vi "GetBeamPrams.vi"(4 "data":dbl[][](array[numeric]) format="%.2f", 7 "ycoords":dbl[](array[numeric]) format="%.2f", 8 "x coords":dbl[](array[numeric]) format="%.2f") -> (0 "3 dB beamwidth (cm)":dbl format="%.4f", 1 "lateral pressure (y)":cluster{"output":dbl[], "output":dbl[]}(graph), 2 "axial peak (cm)":dbl format="%.2f", 3 "axial pressure (z)":cluster{dbl[], "output":dbl[]}(graph))   [LabVIEW 2022 SP3]
uses:
  <vilib>/Utility/file.llb/Read From Spreadsheet File (DBL).vi
  <vilib>/Utility/file.llb/Write To Spreadsheet File (DBL).vi
  <vilib>/Analysis/NI_AALBase.lvlib
panel:
  in  "Case Constant\n(See Context Help)":bool=TRUE
  in  "save main axis":bool
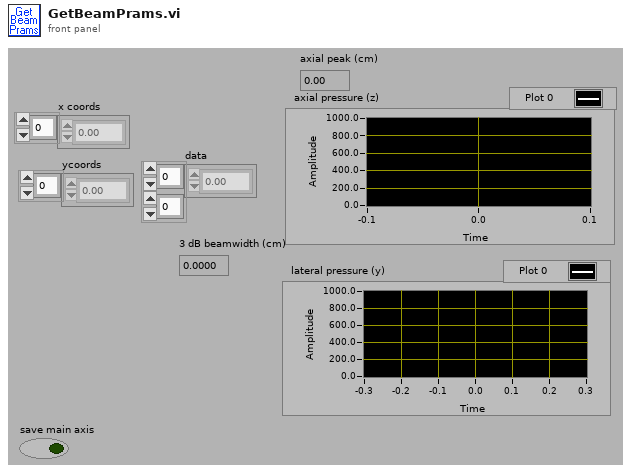
[diagram p1: front panel]
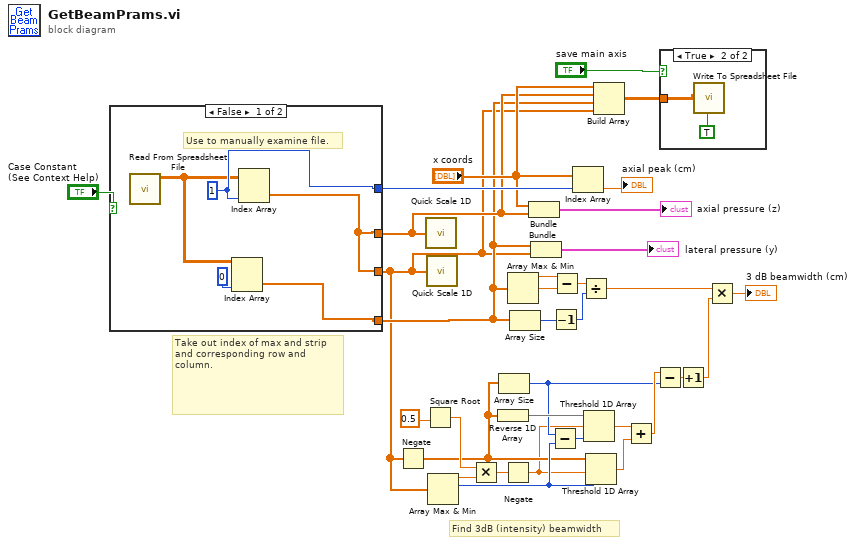
[diagram p0: block diagram]
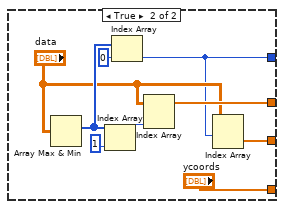
[diagram p3: hidden frame]
diagram:
  # "Take out index of max and strip and corresponding row and column."
  # "Find 3dB (intensity) beamwidth"
  n1 = case shown="False" "Case Constant\n(See Context Help)" {
    tunnel: [w37 w47] -> w5
    tunnel: [w37 w46] -> w3
    tunnel: [w35 w40] -> w10
    tunnel: [w38 "ycoords"] -> w4
    frame False {
      w35 = 1
      # "Use to manually examine file."
      n2 = call-poly <vilib>:"Read From Spreadsheet File.vi"() -> ("all rows"=w34:dbl[][])  [unwired: 4 in, 7 out]
      n3 = Index Array(array=w34, index (col)=0) -> (element=w38:dbl[])  [unwired: 1 in]
      n4 = Index Array(array=w34, index (col)=w35) -> (element=w37:dbl[])  [unwired: 1 in]
    }
    frame True {
      n5 = Array Max & Min(array="data") -> (max index (indices)=w45:i32[])  [unwired: 3 out]
      n6 = Index Array(array=w45, index=1) -> (element=w41:i32)
      n7 = Index Array(array=w45, index=0) -> (element=w40:i32)
      n8 = Index Array(array="data", index (col)=w41) -> (element=w47:dbl[])  [unwired: 1 in]
      n9 = Index Array(array="data", index (row)=w40) -> (element=w46:dbl[])  [unwired: 1 in]
    }
  }
  n10 = Negate(x=w3) -> (-x=w12:dbl[])
  n11 = Square Root(x=0.5) -> (sqrt(x)=w24:dbl)
  n12 = call <vilib>:"Quick Scale 1D.vi"("X"=w5) -> ()  [unwired: 3 out]
  n13 = call <vilib>:"Quick Scale 1D.vi"("X"=w3) -> ()  [unwired: 3 out]
  n14 = Array Max & Min(array=w3) -> (max value=w33:dbl, max index (indices)=w15:i32)  [unwired: 2 out]
  n15 = Multiply(x=w24, y=w33) -> (x*y=w17:dbl)
  n16 = Reverse 1D Array(array=w12) -> (reversed array=w32:dbl[])
  n17 = Array Size(array=w12) -> (size(s)=w13:i32)
  n18 = Negate(x=w17) -> (-x=w11:dbl)
  n19 = Array Max & Min(array=w4) -> (max value=w23:dbl, min value=w22:dbl)  [unwired: 2 out]
  n20 = Array Size(array=w4) -> (size(s)=w20:i32)
  n21 = Bundle("x coords"="x coords", "data"=w5) -> (→"axial pressure (z)":cluster{"x coords":dbl[], "data":dbl[]})  [unwired: 1 out]
  n22 = Bundle("ycoords"=w4, "data"=w3) -> (→"lateral pressure (y)":cluster{"ycoords":dbl[], "data":dbl[]})  [unwired: 1 out]
  n23 = Subtract(x=w13, y=w15) -> (x-y=w16:i32)
  n24 = Decrement(x=w20) -> (x-1=w19:i32)
  n25 = Subtract(x=w23, y=w22) -> (x-y=w21:dbl)
  n26 = Index Array(array="x coords", index=w10) -> (element=→"axial peak (cm)":dbl)
  n27 = Divide(x=w21, y=w19) -> (x/y=w18:dbl)
  n28 = Threshold 1D Array(1:w16, 2:w11, 3:w32) -> (0:w31:dbl)
  n29 = Threshold 1D Array(1:w15, 2:w11, 3:w12) -> (0:w30:dbl)
  n30 = Build Array("x coords", w5, w4, w3) -> (w2:dbl[][])
  n31 = Add(x=w31, y=w30) -> (x+y=w14:dbl)
  n32 = Subtract(x=w14, y=w13) -> (x-y=w9:dbl)
  n33 = case shown="True" "save main axis" {
    tunnel: w2 -> [_ w49]
    frame False {
    }
    frame True {
      n34 = call-poly <vilib>:"Write To Spreadsheet File.vi"("transpose? (no:F)"=TRUE, "2D data"=w49) -> ()  [unwired: 4 in, 3 out]
    }
  }
  n35 = Increment(x=w9) -> (x+1=w8:dbl)
  n36 = Multiply(x=w18, y=w8) -> (x*y=→"3 dB beamwidth (cm)":dbl)
